vi "Create CONNACK Packet.vi"(5 "CONNACK type":refnum<class "CONNACK.lvclass">, 8 "error in (no error)":errorcluster, 10 "Return Code":T1, 11 "Session Present":bool) -> (0 "error out":errorcluster, 2 "Bytes Stream":u8[](array[numeric]) format="%08b", 3 "CONNACK":refnum<class "CONNACK.lvclass">)   [LabVIEW 2013, in "MQTT_Control_Packets.lvlib" / "CONNACK.lvclass"]
uses:
  CONNACK.lvclass
  Connect Return Code -- enum.ctl
  ControlPacket/ControlPacket.lvclass/ControlPacket.ctl
  ControlPacket/ControlPacket.lvclass
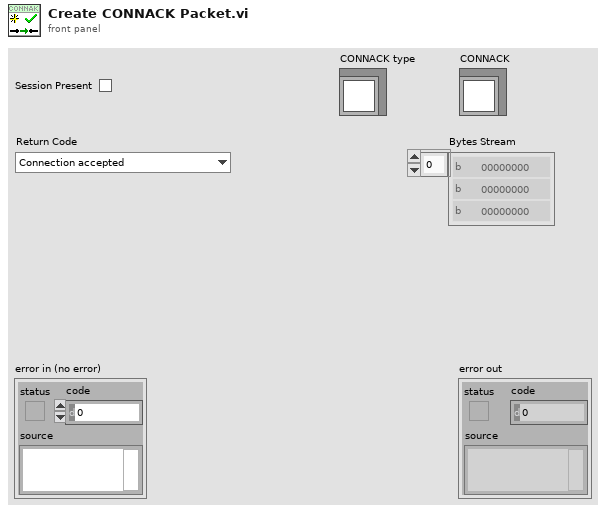
[diagram p1: front panel]
types:
  T1 = typedef "MQTT_Control_Packets.lvlib/CONNACK.lvclass/Connect Return Code -- enum.ctl" = enum16{"Connection accepted", "Unacceptable protocol version", "Identifier Rejected", "Server Unavailable", "Bad Username or Password", "Not Authorized"}
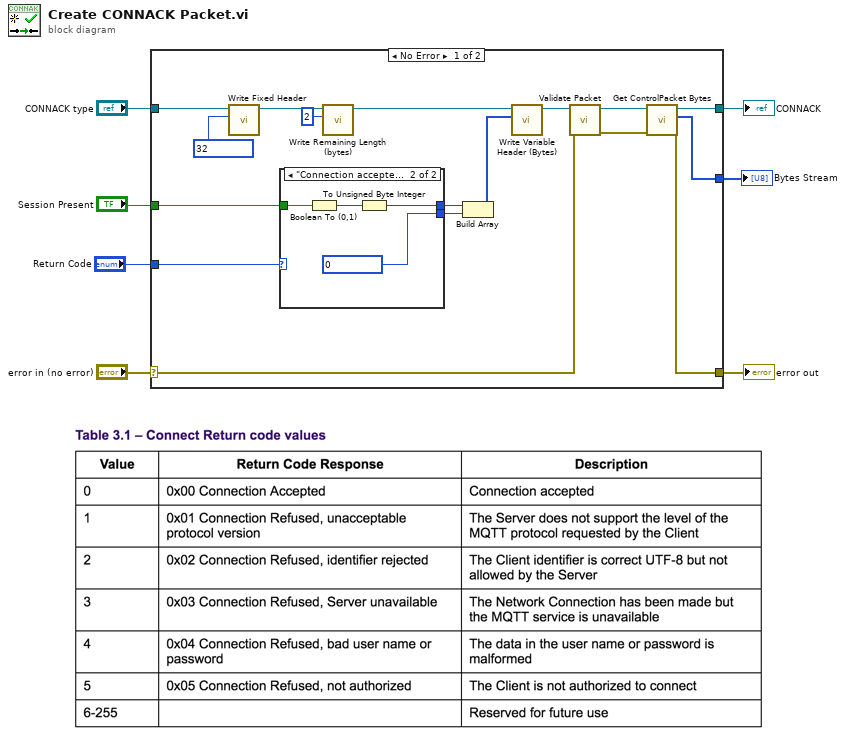
[diagram p0: block diagram]
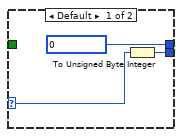
[diagram p2: hidden frame]
diagram:
  n1 = case shown="No Error" "error in (no error)" {
    selector: "error in (no error)" -> [w18 w33]
    tunnel: [w9 w33] -> w6
    tunnel: [w11 w32] -> w4
    tunnel: "CONNACK type" -> [w23 w32]
    tunnel: "Session Present" -> [w16 _]
    tunnel: "Return Code" -> [w17 _]
    tunnel: [w8 _] -> w1
    frame No Error {
      n2 = call "Write Fixed Header.vi"("Fixed Header"=u8 32, "ControlPacket in"=w23) -> ("ControlPacket out"=w15:refnum<class "CONNACK.lvclass">)  [unwired: 9 in]
      n3 = case shown="\"Connection accepted\"" w17 {
        selector: w17 -> [w25 _]
        tunnel: [u8 0 w28] -> w20
        tunnel: [w27 u8 0] -> w19
        tunnel: w16 -> [_ w30]
        frame Default {
          n4 = To Unsigned Byte Integer(number=w25) -> (unsigned 8bit integer=w27:u8)
        }
        frame "Connection accepted" {
          n5 = Boolean To (0,1)(Boolean=w30) -> (0, 1=w29:i16)
          n6 = To Unsigned Byte Integer(number=w29) -> (unsigned 8bit integer=w28:u8)
        }
      }
      n7 = call "Write Remaining Length (bytes).vi"("Remaining Length (bytes)"=u32 2, "ControlPacket in"=w15) -> ("ControlPacket out"=w14:refnum<class "CONNACK.lvclass">)  [unwired: 9 in]
      n8 = Build Array(w20, w19) -> (w22:u8[])
      n9 = call "Write Variable Header (Bytes).vi"("Variable Header (Bytes)"=w22, "ControlPacket in"=w14) -> ("ControlPacket out"=w21:refnum<class "CONNACK.lvclass">)  [unwired: 9 in]
      n10 = call "Validate Packet.vi"("error in (no error)"=w18, "ControlPacket in"=w21) -> ("error out"=w10:errorcluster, "ControlPacket out"=w12:refnum<class "CONNACK.lvclass">)  [unwired: 8 in]
      n11 = call "Get ControlPacket Bytes.vi"("error in (no error)"=w10, "ControlPacket"=w12) -> ("error out"=w9:errorcluster, "Bytes Stream"=w8:u8[], "ControlPacket dup"=w11:refnum<class "CONNACK.lvclass">)  [unwired: 6 in, 1 out]
    }
    frame Error {
    }
  }
  "error out" <- w6
  "CONNACK" <- w4
  "Bytes Stream" <- w1
